vi "CAN Jaguar Open.vi"(6 "Inverted":bool, 8 "error in (no error)":errorcluster, 10 "Control Mode":T2, 11 "Device Number":u8) -> (0 "error out":errorcluster, 3 "CAN Jaguar Ref Out":T1={"Device Number"=0, "Control Mode"=enum."Percent VBus", "Inverted"=FALSE, "Semaphore"=refnum, "Max Vout"=12.0, "DevStatus"={"status"=FALSE, "code"=0, "source"=""}})   [LabVIEW 2009, in "CAN.lvlib"]
uses:
  CAN.lvlib
  SubVIs/CAN Jaguar Control Mode.ctl
  SubVIs/CAN Jaguar Ref.ctl
  SubVIs/CAN Token Message IDs.ctl
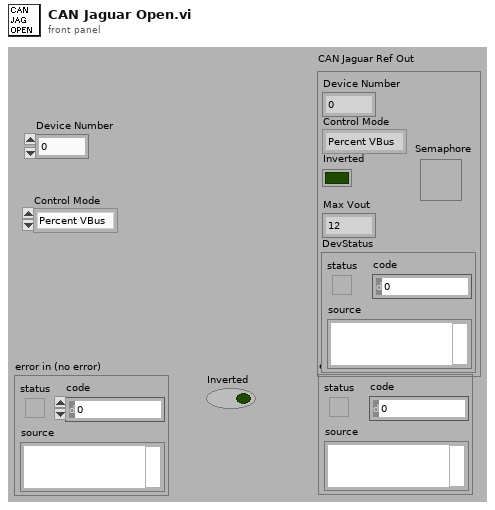
[diagram p1: front panel]
types:
  T1 = typedef "CAN.lvlib/CAN Jaguar Ref.ctl" = cluster{"Device Number":u8, "Control Mode":T2, "Inverted":bool, "Semaphore":T3, "Max Vout":dbl, "DevStatus":errorcluster}
  T2 = typedef "CAN.lvlib/CAN Jaguar Control Mode.ctl" = enum16{"Percent VBus", "Speed", "Position", "Current"}
  T3 = typedef "Semaphore RefNum" = refnum<k1>
  T4 = typedef "CAN.lvlib/CAN Token Message IDs.ctl" = u32
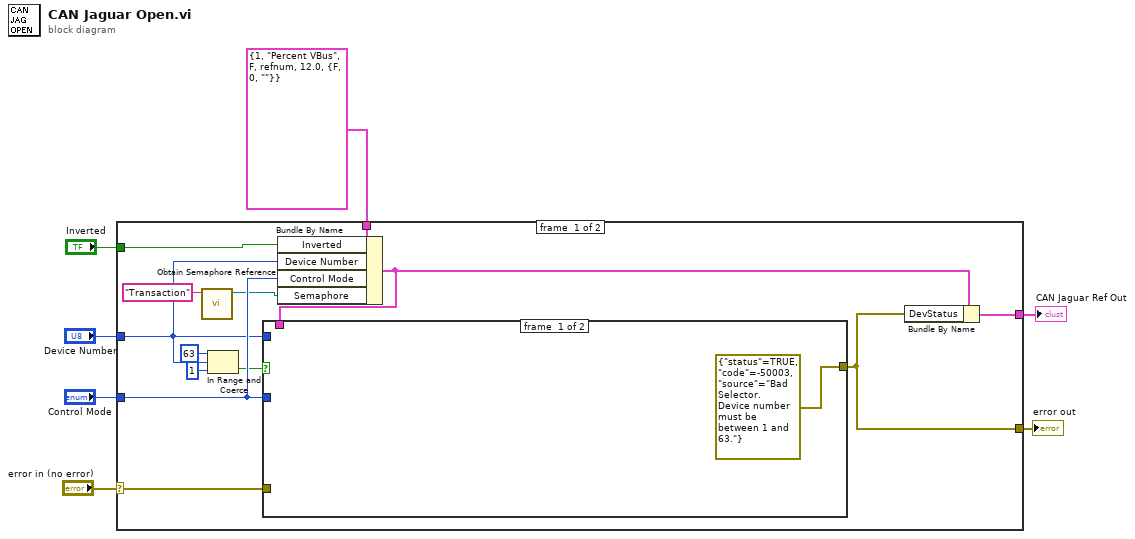
[diagram p0: block diagram]
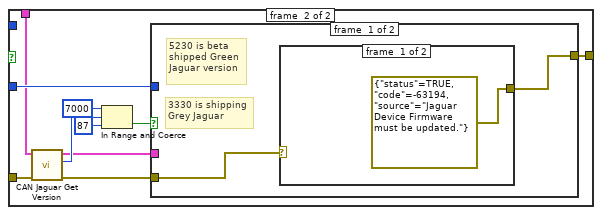
[diagram p2: hidden frame]
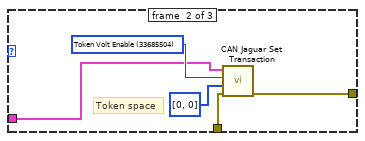
[diagram p5: hidden frame]
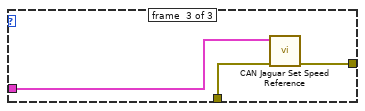
[diagram p6: hidden frame]
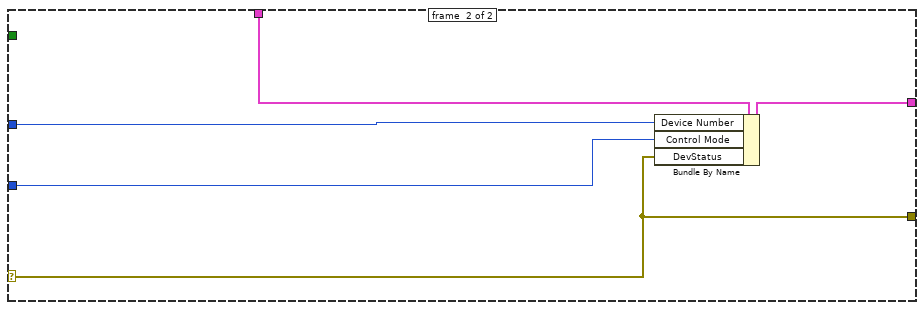
[diagram p7: hidden frame]
diagram:
  n1 = case shown="No Error" "error in (no error)" {
    selector: "error in (no error)" -> [w18 w49]
    tunnel: T1 {"Device Number"=1, "Control Mode"=enum."Percent VBus", "Inverted"=FALSE, "Semaphore"=refnum, "Max Vout"=12.0, "DevStatus"={"status"=FALSE, "code"=0, "source"=""}} ("CAN Jaguar Ref Out") -> [w20 w53]
    tunnel: [w10 w52] -> w6
    tunnel: [w9 w49] -> w5
    tunnel: "Control Mode" -> [w19 w50]
    tunnel: "Device Number" -> [w17 w51]
    tunnel: "Inverted" -> [w13 _]
    frame #0 {
      n2 = call <vilib>:"Obtain Semaphore Reference.vi"("name (unnamed)"="Transaction") -> ("semaphore"=w12:T3)  [unwired: 2 in, 4 out]
      n3 = In Range and Coerce(upper limit=u8 63, x=w17, lower limit=u8 1) -> (In Range?=w14:bool)  [unwired: 1 out]
      n4 = Bundle By Name(cluster=w20, "Inverted"=w13, "Device Number"=w17, "Control Mode"=w19, "Semaphore"=w12) -> (w11:T1)
      n5 = case shown="True" w14 {
        tunnel: [errorcluster {"status"=TRUE, "code"=-50003, "source"="Bad Selector.  Device number must be between 1 and 63."} ("error out") w31] -> w9
        tunnel: w19 -> [_ w30]
        tunnel: w17 -> [_ _]
        tunnel: w18 -> [_ w29]
        tunnel: w11 -> [_ w23]
        frame #0 {
        }
        frame #1 {
          n6 = call "CAN Jaguar Get Version.vi"("error in (no error)"=w29, "CAN Jaguar Ref"=w23) -> ("error out"=w28:errorcluster, "Firmware Version"=w27:u32, "CAN Jaguar Ref Out"=w22:T1)  [unwired: 7 out]
          n7 = In Range and Coerce(upper limit=u32 7000, x=w27, lower limit=u32 87) -> (In Range?=w26:bool)  [unwired: 1 out]
          n8 = case shown="True" w26 {
            tunnel: [w33 w39] -> w31
            tunnel: w30 -> [_ w37]
            tunnel: w28 -> [w32 w38]
            tunnel: w22 -> [_ w36]
            frame #0 {
              # "5230 is beta\nshipped Green\nJaguar version"
              # "3330 is shipping\nGrey Jaguar"
              n9 = case shown="No Error" w32 {
                selector: w32 -> [_ w35]
                tunnel: [errorcluster {"status"=TRUE, "code"=-63194, "source"="Jaguar Device Firmware must be updated."} ("error IO") w35] -> w33
                frame #0 {
                }
                frame #1 {
                }
              }
            }
            frame #1 {
              n10 = case shown="\"Percent VBus\"" w37 {
                tunnel: [w40 w45 w47] -> w39
                tunnel: w38 -> [w40 w44 w46]
                tunnel: w36 -> [_ w41 w48]
                frame #0 {
                }
                frame #1 {
                  w43 = T4 33685504 items=["Token Volt Enable"=33685504, "Token Volt Set"=33685632, "Token Speed Enable"=33686528, "Token Speed Set"=33686656, "Token Position Enable"=33688576, "Token Position Set"=33688704, "Token Current Enable"=33689600, "Token Current Set"=33689728] ("CAN Token Message IDs")
                  # "Token space"
                  n11 = call "CAN Jaguar Set Transaction.vi"("error in"=w44, "Data"=u8[] [0, 0] ("data"), "Message ID"=w43, "CAN Jaguar Ref"=w41) -> ("error out"=w45:errorcluster)  [unwired: 7 out]
                }
                frame #2 {
                  n12 = call "CAN Jaguar Set Speed Reference.vi"("error in (no error)"=w46, "CAN Jaguar Ref"=w48) -> ("error out"=w47:errorcluster)  [unwired: 1 in, 8 out]
                }
              }
            }
          }
        }
      }
      n13 = Bundle By Name(cluster=w11, "DevStatus"=w9) -> (w10:T1)
    }
    frame #1 {
      n14 = Bundle By Name(cluster=w53, "Device Number"=w51, "Control Mode"=w50, "DevStatus"=w49) -> (w52:T1)
    }
  }
  "error out" <- w5
  "CAN Jaguar Ref Out" <- w6
